vi "idn_action.vi"(0 "HGF_ImaqUsb":refnum<class "HGF_ImaqUsb.lvclass">, 5 "error in (no error)":errorcluster) -> (12 "resourceString":string, 13 "additionalInfo":string, 14 "HGF_ImaqUsb out":refnum<class "HGF_ImaqUsb.lvclass">, 15 "driverRevision":string="unknown", 16 "firmwareRevision":string="unknown", 17 "vendor":string="unknown", 18 "model":string="unknown", 19 "error out":errorcluster)   [LabVIEW 2009, in "HGF_ImaqUsb.lvclass"]
doc: "This VI queries the current instrument firmware revision and instrument driver revision.\n\nFor detailed driver information including modification history, refer to the Readme file.\n\n<b>Hint:</b> This is a dynamic dispatch VI to be implemented by child classes."
uses:
  HGF_ImaqUsb.lvclass
  HGF_IMAQDevice/HGF_IMAQDevice.lvclass
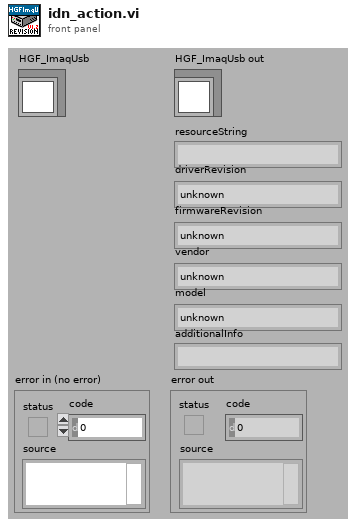
[diagram p1: front panel]
types:
  T1 = cluster{"Major":u16, "Minor":u16, "Fix":u16, "Build":u16}
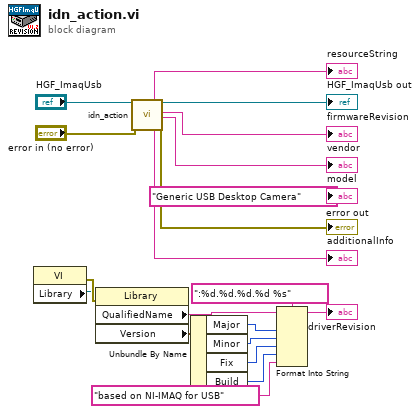
[diagram p0: block diagram]
diagram:
  n1 = property class="VI"() -> (error out=w14:errorcluster, "Library"=w11:refnum<vi>)  [unwired: 2 in, 1 out]
  n2 = property class="Library"(reference=w11, error in=w14) -> ("QualifiedName"=w13:string, "Version"=w5:T1)  [unwired: 2 out]
  n3 = call-parent "idn_action.vi"("HGF_IMAQDevice"="HGF_ImaqUsb", "error in (no error)"="error in (no error)") -> ("resourceString"=→"resourceString":string, "additionalInfo"=→"additionalInfo":string, "HGF_IMAQDevice out"=→"HGF_ImaqUsb out":refnum<class "HGF_ImaqUsb.lvclass">, "firmwareRevision"=→"firmwareRevision":string, "vendor"=→"vendor":string, "error out"=→"error out":errorcluster)  [unwired: 12 out]
  n4 = Unbundle By Name(w5) -> ("Major"=w6:u16, "Minor"=w7:u16, "Fix"=w8:u16, "Build"=w9:u16)
  n5 = Format Into String(format string=":%d.%d.%d.%d %s", initial string=w13, w6, w7, w8, w9, "based on NI-IMAQ for USB" ("driverRevision")) -> (resulting string=→"driverRevision":string)  [unwired: 1 in, 1 out]
  "model" <- "Generic USB Desktop Camera" ("model")
